vi "PH_PILS.set Radiation Shutters.vi"(0 "i ref in":refnum<vi>, 5 "error in":errorcluster) -> (14 "i ref out":refnum<vi>, 19 "error out":errorcluster)   [LabVIEW 2014, in "PH_PILS.lvlib"]
doc: "This VI calculates and indicatzes the state of the radiation safety shutters."
uses:
  PH_PILS.lvlib
  PH_Common/PH_Common.lvlib
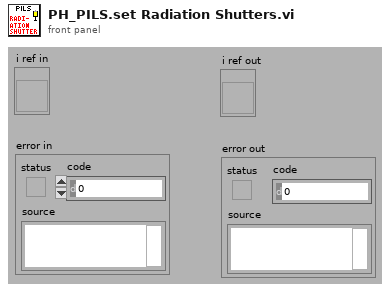
[diagram p1: front panel]
types:
  T1 = typedef "PH_PILS.lvlib/PH_PILS.i attribute.ctl" = cluster{"Boolean":cluster{"GUI Ref":refnum<vi>, "Status":i32}[], "GUI Refs Exp. Shutters":cluster{"1":refnum<vi>, "2":refnum<vi>, "3":refnum<vi>, "4":refnum<vi>}, "Tristate2Run GUI Refs":refnum<vi>[], "EO-Likes":cluster{"GUI Ref":refnum<vi>, "Status":i32}[], "Operation Mode":cluster{"Operation Mode":T2, "GUI":cluster{"Ref State":refnum<vi>, "Ref":refnum<vi>}, "Servicemode":cluster{"Tagname":string, "Status":i32}, "Labormode":cluster{"Tagname":string, "Status":i32}, "Searchmode":cluster{"Tagname":string, "Status":i32}, "Shotmode":cluster{"Tagname":string, "Status":i32}}, "Submode":cluster{"Submode":T3, "GUI":cluster{"Ref State":refnum<vi>, "Ref":refnum<vi>}, "Submode":cluster{"Tagname":string, "Status":i32}}, "Experiment":cluster{"Experiment":enum16{"unknown", "intern", "4 (Z6)", "3", "2", "1"}, "GUI":cluster{"Ref State":refnum<vi>, "Ref":refnum<vi>}, "intern":cluster{"Tagname":string, "Status":i32}, "Exp 4":cluster{"Tagname":string, "Status":i32}, "Exp 3":cluster{"Tagname":string, "Status":i32}, "Exp 2":cluster{"Tagname":string, "Status":i32}, "Exp 1":cluster{"Tagname":string, "Status":i32}}, "TristateNormal":cluster{"GUI Ref":refnum<vi>, "Status":i32}[], "Door Tags":cluster{"GUI Ref":refnum<vi>, "Status":i32}[], "GUIlessTags":cluster{"Name":string, "Status":i32}[], "Beamline GUI Refs":refnum<vi>[], "Special Boolean":cluster{"GUI Ref":refnum<vi>, "Status":i32}[], "Laserpower":cluster{"GUI Ref":refnum<vi>, "Status":i32}[], "Shutter":cluster{"GUI Ref":refnum<vi>, "Status":i32}[], "Tristate EO Like":cluster{"GUI Ref":refnum<vi>, "Status":i32}[], "PP":cluster{"GUI Ref":refnum<vi>, "Status":i32, "Head Ref":refnum<vi>, "Slider Ref":refnum<vi>}[], "Switch Knobs":cluster{"GUI Ref":refnum<vi>, "Status":i32}[], "Latch Knob GUI Refs":refnum<vi>[], "FailureCounter":i32, "Enabled Status":cluster{"Laser":i32, "PreAmp":i32, "MainAmp":i32}, "Mercury":refnum<vi>, "Instance Rods":string, "Logfile":path, "Beckhoff-Instance Internal":string, "Beckhoff-Instance External":string, "Enabling Rights":cluster{"Name":string, "Password":string, "PA?":bool, "MA?":bool, "Exp?":bool}[]}
  T2 = typedef "PH_PILS.lvlib/PH_PILS.Operation Mode.ctl" = enum16{"unknown", "Service", "Labor", "Search", "Shot"}
  T3 = typedef "PH_PILS.lvlib/PH_PILS.Submode.ctl" = enum16{"unknown", "HV-Normal", "HV-Test"}
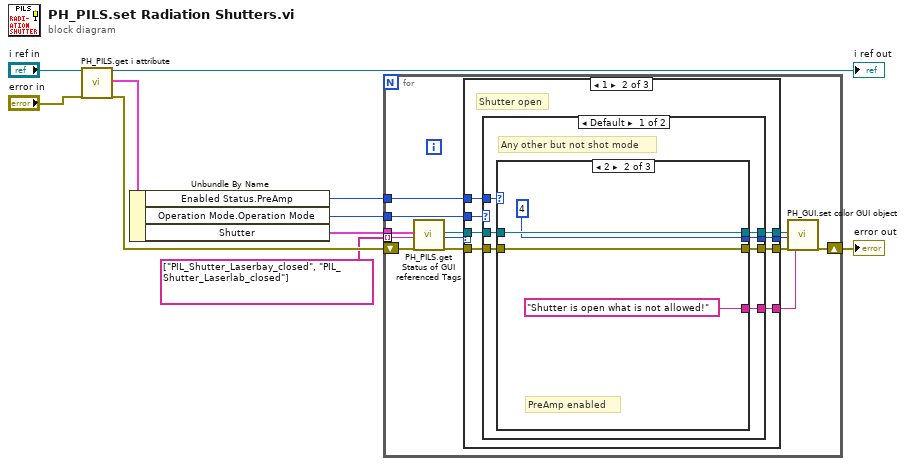
[diagram p0: block diagram]
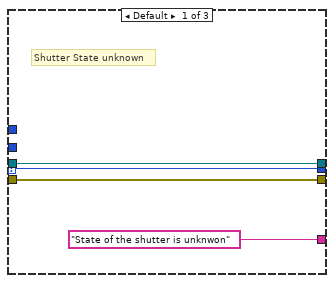
[diagram p2: hidden frame]
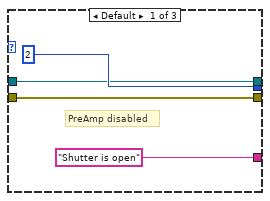
[diagram p3: hidden frame]
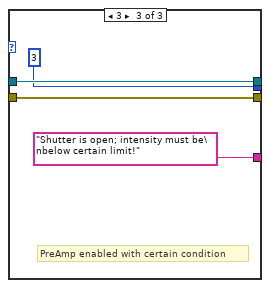
[diagram p4: hidden frame]
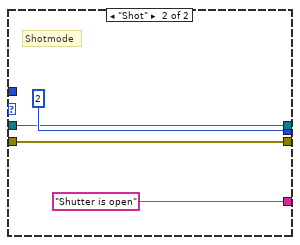
[diagram p5: hidden frame]
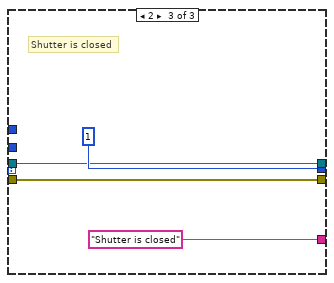
[diagram p6: hidden frame]
diagram:
  n1 = call "PH_PILS.get i attribute.vi"("i ref in"="i ref in", "error in (no error)"="error in") -> ("i ref out"=→"i ref out":refnum<vi>, "i attribute"=w7:T1, "error out"=w5:errorcluster)  [unwired: 15 in]
  n2 = Unbundle By Name(w7) -> ("Enabled Status.PreAmp"=w1:i32, "Operation Mode.Operation Mode"=w2:T2, "Shutter"=w6:cluster{"GUI Ref":refnum<vi>, "Status":i32}[])
  n3 = for {
    tunnel: w6 -> [w23]
    shift-right: [w21] -> w4
    shift-left: w5 -> [w22]
    tunnel: string[] ["PIL_Shutter_Laserbay_closed", "PIL_Shutter_Laserlab_closed"] -> [w20] mode=indexing
    tunnel: w2 -> [w17]
    tunnel: w1 -> [w16]
    n4 = call "PH_PILS.get Status of GUI referenced Tags.vi"("Tags"=w23, "Tagname"=w20, "error in"=w22) -> ("GUI Ref"=w13:refnum<vi>, "Status"=w19:i32, "error out"=w15:errorcluster)  [unwired: 13 in, 1 out]
    n5 = case shown="1" w19 {
      selector: w19 -> [w27 _ _]
      tunnel: [w27 w33 1 ("Status")] -> w18
      tunnel: w17 -> [_ w35 _]
      tunnel: w16 -> [_ w34 _]
      tunnel: w15 -> [w26 w32 w61]
      tunnel: [w26 w31 w61] -> w14
      tunnel: w13 -> [w25 w29 w60]
      tunnel: [w25 w30 w60] -> w12
      tunnel: ["State of the shutter is unknwon" w28 "Shutter is closed"] -> w11
      frame Default {
        # "Shutter State unknown"
      }
      frame 1 {
        # "Shutter open"
        n6 = case shown="Default" w35 {
          tunnel: [w41 2] -> w33
          tunnel: w34 -> [w42 _]
          tunnel: w32 -> [w40 w57]
          tunnel: [w39 w57] -> w31
          tunnel: [w37 w56] -> w30
          tunnel: w29 -> [w38 w56]
          tunnel: [w36 "Shutter is open"] -> w28
          frame Default {
            # "Any other but not shot mode"
            n7 = case shown="2" w42 {
              tunnel: [2 4 3] -> w41
              tunnel: w40 -> [w45 w49 w53]
              tunnel: [w45 w49 w53] -> w39
              tunnel: w38 -> [w44 w50 w54]
              tunnel: [w44 w50 w54] -> w37
              tunnel: ["Shutter is open" "Shutter is open what is not allowed!" "Shutter is open; intensity must be\nbelow certain limit!"] -> w36
              frame Default {
                # "PreAmp disabled"
              }
              frame 2 {
                # "PreAmp enabled"
              }
              frame 3 {
                # "PreAmp enabled with certain condition"
              }
            }
          }
          frame "Shot" {
            # "Shotmode"
          }
        }
      }
      frame 2 {
        # "Shutter is closed"
      }
    }
    n8 = call "PH_GUI.set color GUI object.vi"("GUI object Ref"=w12, "State"=w18, "error in (no error)"=w14, "Tip Strip (N/A)"=w11) -> ("error out"=w21:errorcluster)  [unwired: 15 in]
  }
  "error out" <- w4
